vi "NotARefNumBase.vi"(3 "reference in":refnum<class "G#RealTimeTemplate.lvclass">) -> (0 "not a refnum?":bool, 1 "reference out":refnum<class "G#RealTimeTemplate.lvclass">)   [LabVIEW 2020, in "G#RealTimeTemplate.lvclass"]
doc: "Checks if the specified object reference is valid."
uses:
  G#RealTimeTemplate.lvclass
  ObjectAttributesRef.ctl
  protected/ObjectAttributes.ctl
  G#RealTimeTemplate.lvclass/G#RealTimeTemplate.ctl
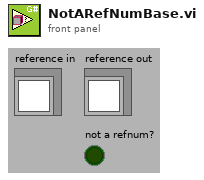
[diagram p1: front panel]
types:
  T1 = typedef "G#RealTimeTemplate.lvclass/ObjectAttributesRef.ctl" = refnum<data-value>
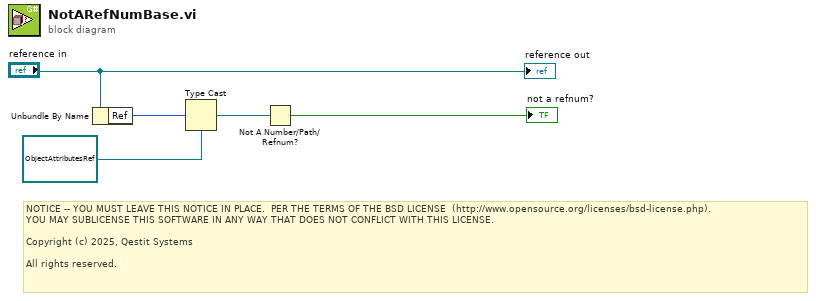
[diagram p0: block diagram]
diagram:
  # "NOTICE -- YOU MUST LEAVE THIS NOTICE IN PLACE.  PER THE TERMS OF THE BSD LICENSE  (http://www.opensource.org/licenses/bsd-license.php).\nYOU MAY SUBLICENSE THIS SOFTWARE IN ANY WAY THAT DOES NOT CONFLICT WITH THIS LICENSE.\n\nCopyright (c) 2025, Qestit Systems\n\nAll rights reserved."
  n1 = Unbundle By Name("reference in") -> ("Ref"=w4:u32)
  n2 = Type Cast(type=T1 refnum ("attributes ref"), x=w4) -> (*(type *) &x=w3:T1)
  n3 = Not A Number/Path/Refnum?(number/path/refnum=w3) -> (NaN/Path/Refnum?=→"not a refnum?":bool)
  "reference out" <- "reference in"
